vi "UpdateMetricCache.vi"(8 "error in (no error)":errorcluster, 9 "Metrics":variant, 11 "MetricDefinitionInstances":T1[](array[typedef])) -> (0 "error out":errorcluster, 1 "Metrics out":variant)   [LabVIEW 2017, in "AnalysisHelper.lvlib"]
uses:
  <vilib>/addons/InsightCM/Utilities/Analysis/Shared/AnalysisHelper.lvlib
  <vilib>/addons/InsightCM/MessageBus/Base/controls/MetricDefinitionInstance.ctl
  <vilib>/addons/InsightCM/MessageBus/Base/controls/KeyValuePair.ctl
  <vilib>/addons/InsightCM/Utilities/Analysis/Shared/controls/BandDomain.ctl
  <vilib>/addons/InsightCM/Utilities/Analysis/Shared/controls/BandCalculation.ctl
  <vilib>/addons/InsightCM/Utilities/PropertyHelpers/PropertyHelpers.lvlib
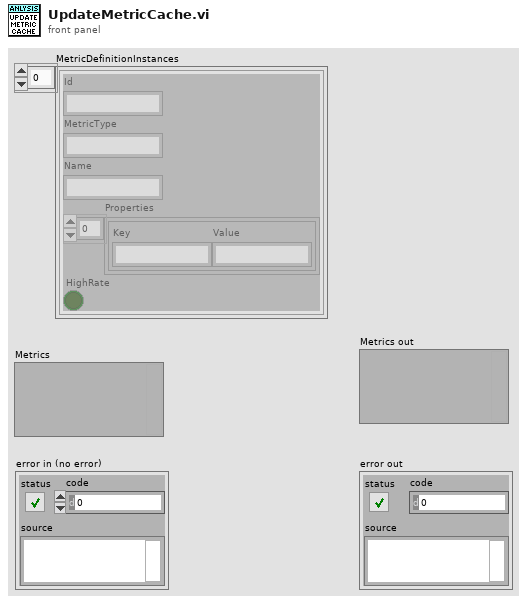
[diagram p1: front panel]
types:
  T1 = typedef "MetricDefinitionInstance.ctl" = cluster{"Id":string, "MetricType":string, "Name":string, "Properties":T2[], "HighRate":bool}
  T2 = typedef "KeyValuePair.ctl" = cluster{"Key":string, "Value":string}
  T3 = typedef "AnalysisHelper.lvlib/BandDomain.ctl" = enum16{"Frequency", "CPM", "Orders"}
  T4 = typedef "AnalysisHelper.lvlib/BandCalculation.ctl" = enum16{"Total", "Max", "Phase"}
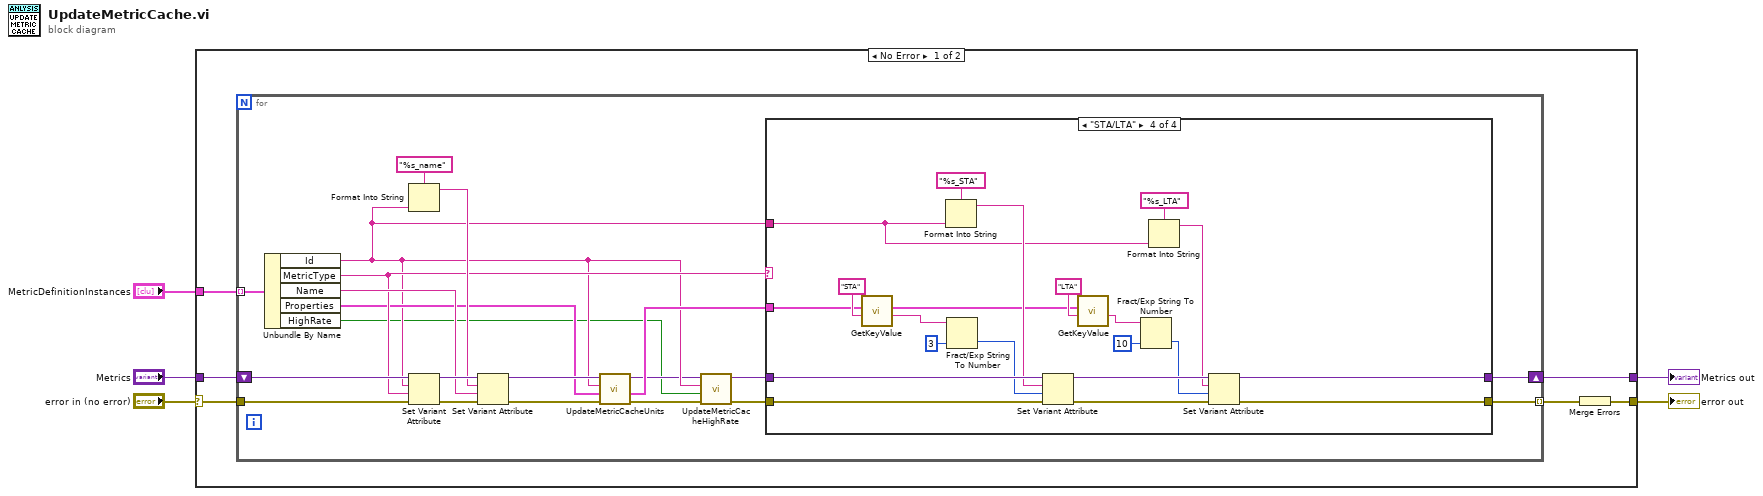
[diagram p0: block diagram]
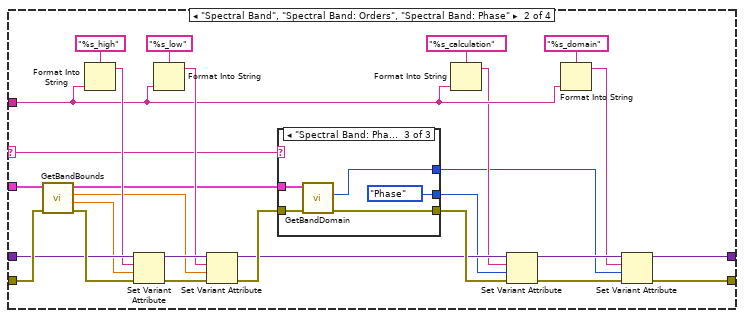
[diagram p3: hidden frame]
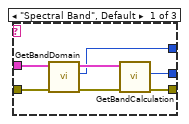
[diagram p4: hidden frame]
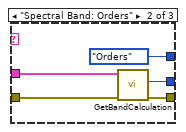
[diagram p5: hidden frame]
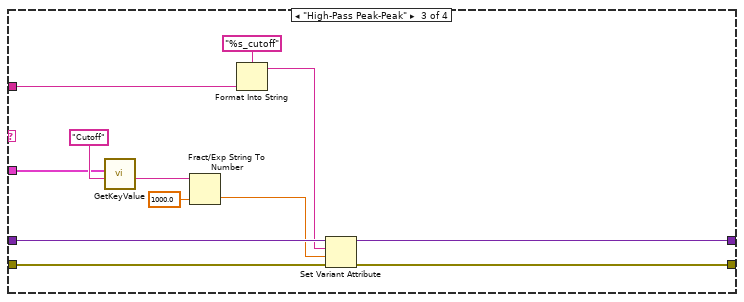
[diagram p6: hidden frame]
diagram:
  n1 = case shown="No Error" "error in (no error)" {
    selector: "error in (no error)" -> [w6 w114]
    tunnel: [w11 w114] -> w5
    tunnel: [w10 w113] -> w4
    tunnel: "Metrics" -> [w9 w113]
    tunnel: "MetricDefinitionInstances" -> [w7 _]
    frame No Error {
      n2 = for {
        tunnel: w7 -> [w32] mode=indexing
        tunnel: w6 -> [w31]
        shift-right: [w28] -> w10
        shift-left: w9 -> [w30]
        tunnel: [w29] -> w8 mode=indexing
        n3 = Unbundle By Name(w32) -> ("Id"=w17:string, "MetricType"=w22:string, "Name"=w23:string, "Properties"=w19:T2[], "HighRate"=w12:bool)
        n4 = Format Into String(format string="%s_name", w17) -> (resulting string=w24:string)  [unwired: 2 in, 1 out]
        n5 = Set Variant Attribute(Variant=w30, name=w17, value=w22, error in=w31) -> (Variant out=w26:variant, error out=w27:errorcluster)  [unwired: 1 out]
        n6 = Set Variant Attribute(Variant=w26, name=w24, value=w23, error in=w27) -> (Variant out=w20:variant, error out=w21:errorcluster)  [unwired: 1 out]
        n7 = call <vilib>:"UpdateMetricCacheUnits.vi"("error in (no error)"=w21, "properties"=w19, "metric definition instance id"=w17, "metric cache in"=w20) -> ("error out"=w16:errorcluster, "properties out"=w18:T2[], "metric cache out"=w14:variant)  [unwired: 5 in]
        n8 = call <vilib>:"UpdateMetricCacheHighRate.vi"("error in (no error)"=w16, "HighRate"=w12, "metric definition instance id"=w17, "metric cache in"=w14) -> ("error out"=w15:errorcluster, "metric cache out"=w13:variant)  [unwired: 6 in]
        n9 = case shown="\"STA/LTA\"" w22 {
          selector: w22 -> [_ w49 _ _]
          tunnel: [w33 w42 w86 w101] -> w29
          tunnel: w15 -> [w33 w60 w80 w104]
          tunnel: [w34 w41 w87 w100] -> w28
          tunnel: w13 -> [w34 w58 w91 w112]
          tunnel: w18 -> [_ w62 w84 w108]
          tunnel: w17 -> [_ w45 w88 w94]
          frame Default {
          }
          frame "Spectral Band", "Spectral Band: Orders", "Spectral Band: Phase" {
            n10 = call <vilib>:"GetBandBounds.vi"("error in (no error)"=w60, "Properties In"=w62) -> ("error out"=w59:errorcluster, "High"=w56:sgl, "Low"=w51:sgl, "Properties Out"=w48:T2[])  [unwired: 6 in]
            n11 = Format Into String(format string="%s_high", w45) -> (resulting string=w53:string)  [unwired: 2 in, 1 out]
            n12 = Set Variant Attribute(Variant=w58, name=w53, value=w56, error in=w59) -> (Variant out=w57:variant, error out=w61:errorcluster)  [unwired: 1 out]
            n13 = Format Into String(format string="%s_low", w45) -> (resulting string=w52:string)  [unwired: 2 in, 1 out]
            n14 = Set Variant Attribute(Variant=w57, name=w52, value=w51, error in=w61) -> (Variant out=w39:variant, error out=w50:errorcluster)  [unwired: 1 out]
            n15 = case shown="\"Spectral Band: Phase\"" w49 {
              tunnel: w50 -> [w69 w71 w78]
              tunnel: w48 -> [w68 w72 w76]
              tunnel: [w65 w74 w77] -> w44
              tunnel: [w64 w73 BandCalculation."Phase" ("Calculation")] -> w38
              tunnel: [w63 BandDomain."Orders" ("Domain") w75] -> w36
              frame "Spectral Band", Default {
                n16 = call <vilib>:"GetBandDomain.vi"("error in (no error)"=w69, "Properties In"=w68) -> ("error out"=w66:errorcluster, "Domain"=w63:T3, "Properties Out"=w67:T2[])  [unwired: 7 in]
                n17 = call <vilib>:"GetBandCalculation.vi"("error in (no error)"=w66, "Properties In"=w67) -> ("error out"=w65:errorcluster, "Calculation"=w64:T4)  [unwired: 7 in, 1 out]
              }
              frame "Spectral Band: Orders" {
                n18 = call <vilib>:"GetBandCalculation.vi"("error in (no error)"=w71, "Properties In"=w72) -> ("error out"=w74:errorcluster, "Calculation"=w73:T4)  [unwired: 7 in, 1 out]
              }
              frame "Spectral Band: Phase" {
                n19 = call <vilib>:"GetBandDomain.vi"("error in (no error)"=w78, "Properties In"=w76) -> ("error out"=w77:errorcluster, "Domain"=w75:T3)  [unwired: 7 in, 1 out]
              }
            }
            n20 = Format Into String(format string="%s_calculation", w45) -> (resulting string=w37:string)  [unwired: 2 in, 1 out]
            n21 = Set Variant Attribute(Variant=w39, name=w37, value=w38, error in=w44) -> (Variant out=w40:variant, error out=w43:errorcluster)  [unwired: 1 out]
            n22 = Format Into String(format string="%s_domain", w45) -> (resulting string=w35:string)  [unwired: 2 in, 1 out]
            n23 = Set Variant Attribute(Variant=w40, name=w35, value=w36, error in=w43) -> (Variant out=w41:variant, error out=w42:errorcluster)  [unwired: 1 out]
          }
          frame "High-Pass Peak-Peak" {
            n24 = call <vilib>:"GetKeyValue.vi"("key"="Cutoff", "key value pairs"=w84) -> ("value"=w82:string)  [unwired: 7 in, 2 out]
            n25 = Fract/Exp String To Number(string=w82, default (0 dbl)=sgl 1000.0 ("default (0 DBL)")) -> (number=w81:sgl)  [unwired: 2 in, 1 out]
            n26 = Format Into String(format string="%s_cutoff", w88) -> (resulting string=w89:string)  [unwired: 2 in, 1 out]
            n27 = Set Variant Attribute(Variant=w91, name=w89, value=w81, error in=w80) -> (Variant out=w87:variant, error out=w86:errorcluster)  [unwired: 1 out]
          }
          frame "STA/LTA" {
            n28 = call <vilib>:"GetKeyValue.vi"("key"="STA", "key value pairs"=w108) -> ("value"=w106:string, "key value pairs out"=w98:T2[])  [unwired: 7 in, 1 out]
            n29 = Format Into String(format string="%s_STA", w94) -> (resulting string=w110:string)  [unwired: 2 in, 1 out]
            n30 = Fract/Exp String To Number(string=w106, default (0 dbl)=3 ("default (0 DBL)")) -> (number=w105:i32)  [unwired: 2 in, 1 out]
            n31 = Set Variant Attribute(Variant=w112, name=w110, value=w105, error in=w104) -> (Variant out=w103:variant, error out=w102:errorcluster)  [unwired: 1 out]
            n32 = call <vilib>:"GetKeyValue.vi"("key"="LTA", "key value pairs"=w98) -> ("value"=w96:string)  [unwired: 7 in, 2 out]
            n33 = Fract/Exp String To Number(string=w96, default (0 dbl)=10 ("default (0 DBL)")) -> (number=w92:i32)  [unwired: 2 in, 1 out]
            n34 = Format Into String(format string="%s_LTA", w94) -> (resulting string=w93:string)  [unwired: 2 in, 1 out]
            n35 = Set Variant Attribute(Variant=w103, name=w93, value=w92, error in=w102) -> (Variant out=w100:variant, error out=w101:errorcluster)  [unwired: 1 out]
          }
        }
      }
      n36 = Merge Errors(w8) -> (w11:errorcluster)
    }
    frame Error {
    }
  }
  "error out" <- w5
  "Metrics out" <- w4
